vi "DANTE acquire single.vi"(0 "Acq in progress":refnum<vi>, 1 "Single Spectrum":refnum<vi>, 6 "Number of boards in chain":u8(slide)=1 scale=1.0..8.0, 8 "Pause button":refnum<vi>, 9 "Acquisition time [s]":dbl=10.0 min=1.0 max=1000.0, 10 "Stop Button":refnum<vi>, 11 "identifier out":string) -> (2 "stats out":T1, 3 "single spectrum":dbl[](array[numeric]))   [LabVIEW 2015]
uses:
  StateTypeDef.ctl
  XGL_DPP.lvlib
panel:
  in  "Stop Acq":bool
  out "Boards to configure":u8(slide) scale=0.0..8.0
  out "spectra to read 3":i64=10
  out "spectra to read":i64=1
  out "spectra":u16[][](array[numeric])
  out "adv stats":u64[][](array[numeric])
  out "Statistics":dbl[][](array[numeric])
  out "State 2":T2=enum."Close library"
  in  "Map points":u32=10
  in  "Time per spectrum [ms]":u32=10 min=1 max=1000000
  in  "Add IP":bool
  out "Acq. in progress":bool
  out "Library Initialized":bool
  in  "Get connected":bool
  in  "Init":bool
  in  "Clear":bool
  in  "Close":bool
  in  "Start acq":bool
  out "Error code":i32
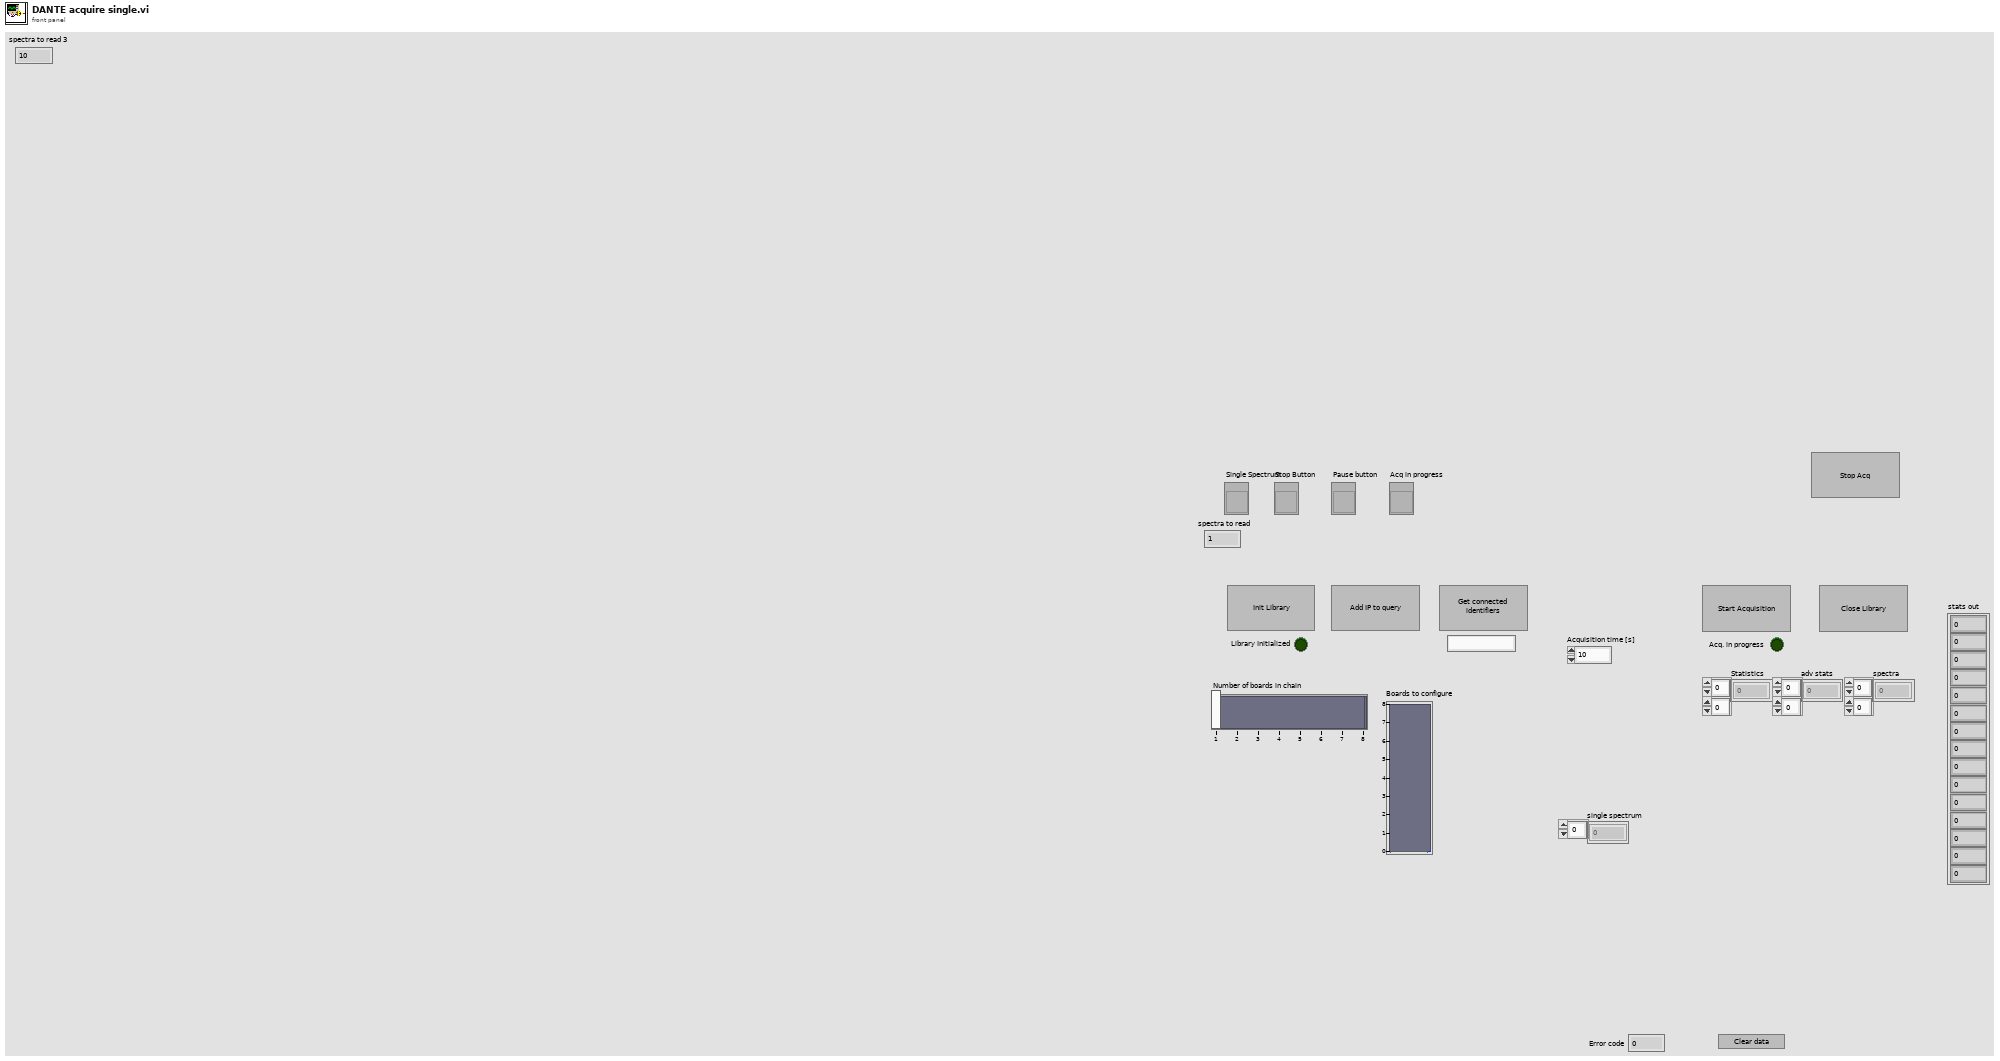
[diagram p1: front panel]
types:
  T1 = cluster{u64, u64, dbl, dbl, u32, u32, u32, u32, u32, u32, u32, u32, u32, u32, u32}
  T2 = typedef "StateTypeDef.ctl" = enum16{"Stop", "Check downloaded spectra", "Get all data", "Read acq mode", "Send running/Get Data", "Add IP to query", "Get serial", "Close library", "Clear", "Acquisition start", "Initialization", "Check Answer", "Configuring", "Wait Answer", "Start map", "Wait input"}
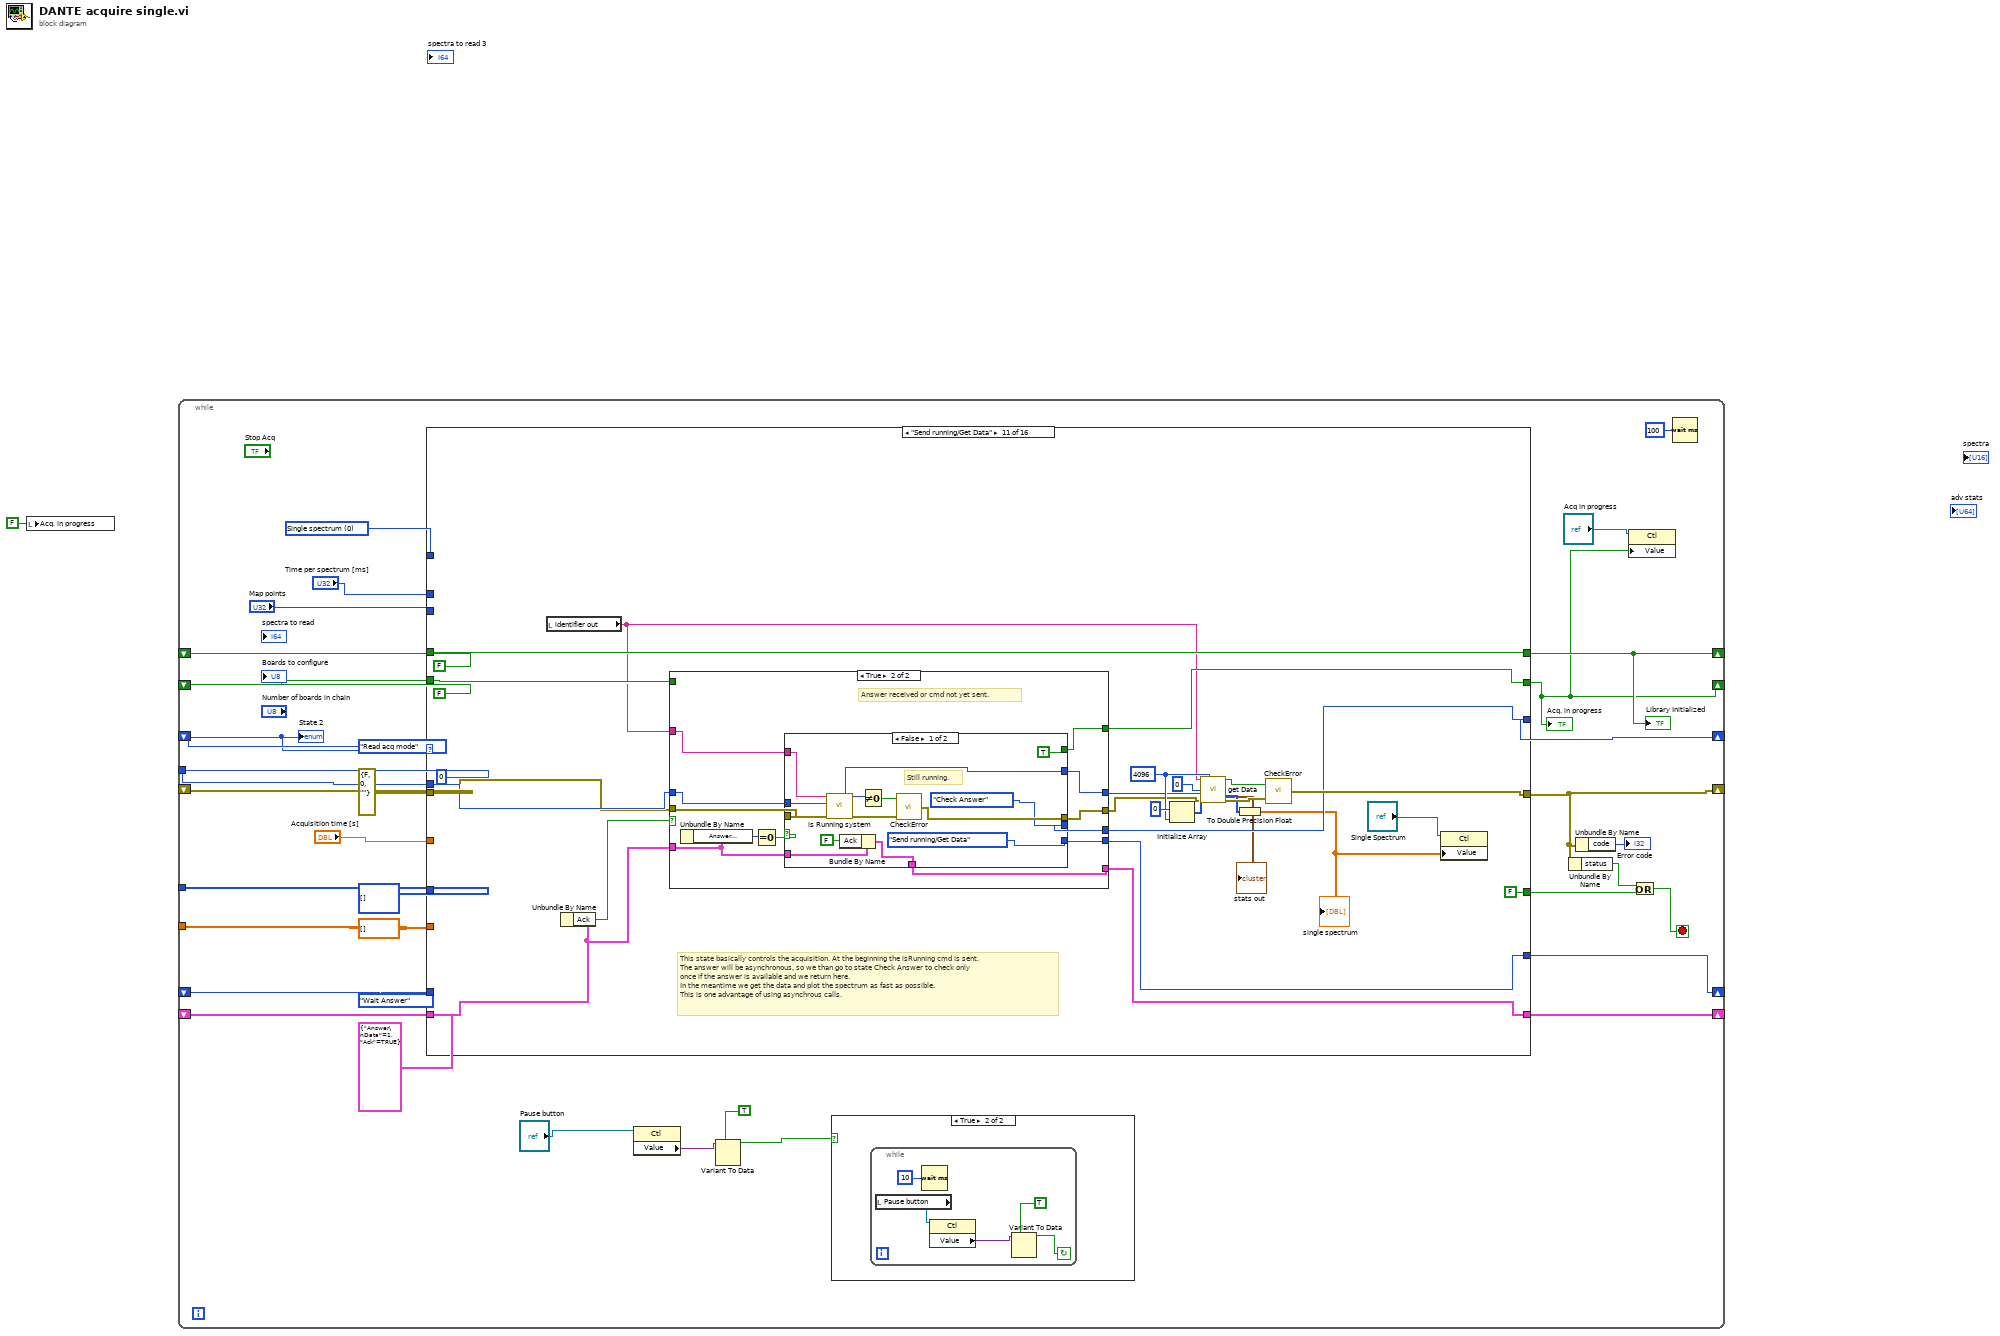
[diagram p0: block diagram]
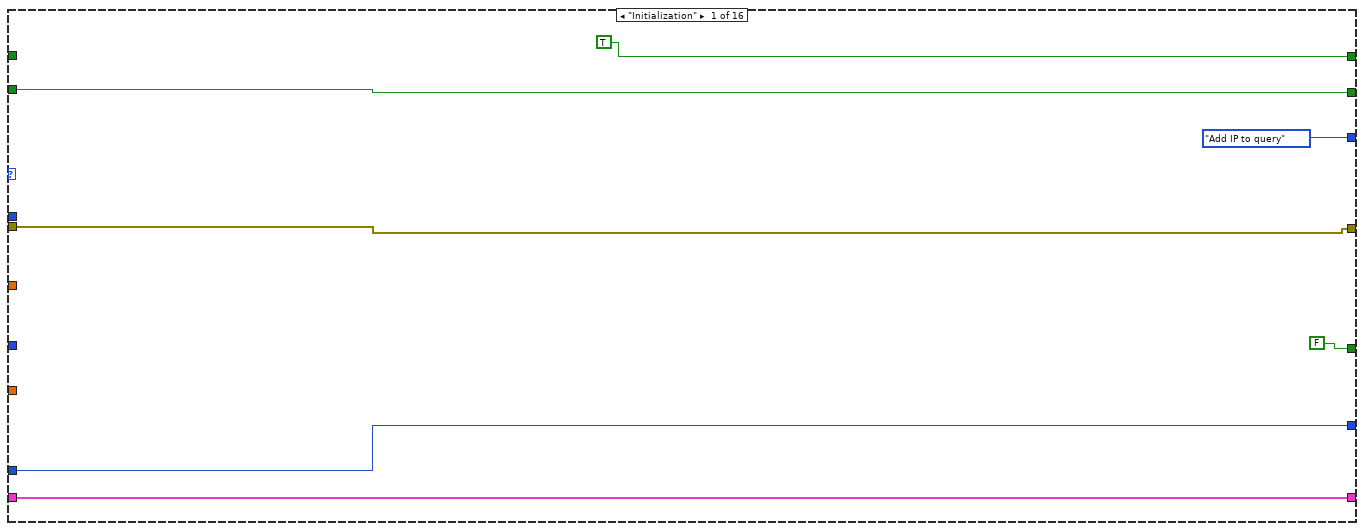
[diagram p3: hidden frame]
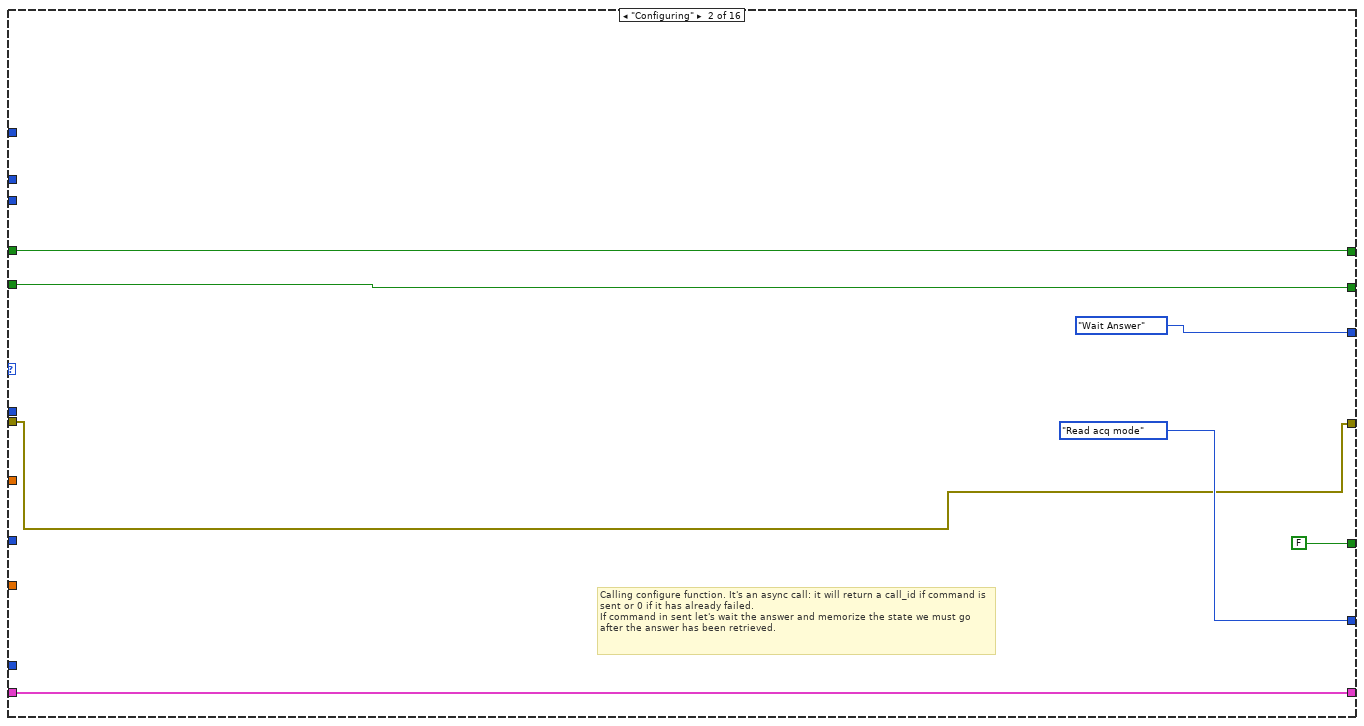
[diagram p4: hidden frame]
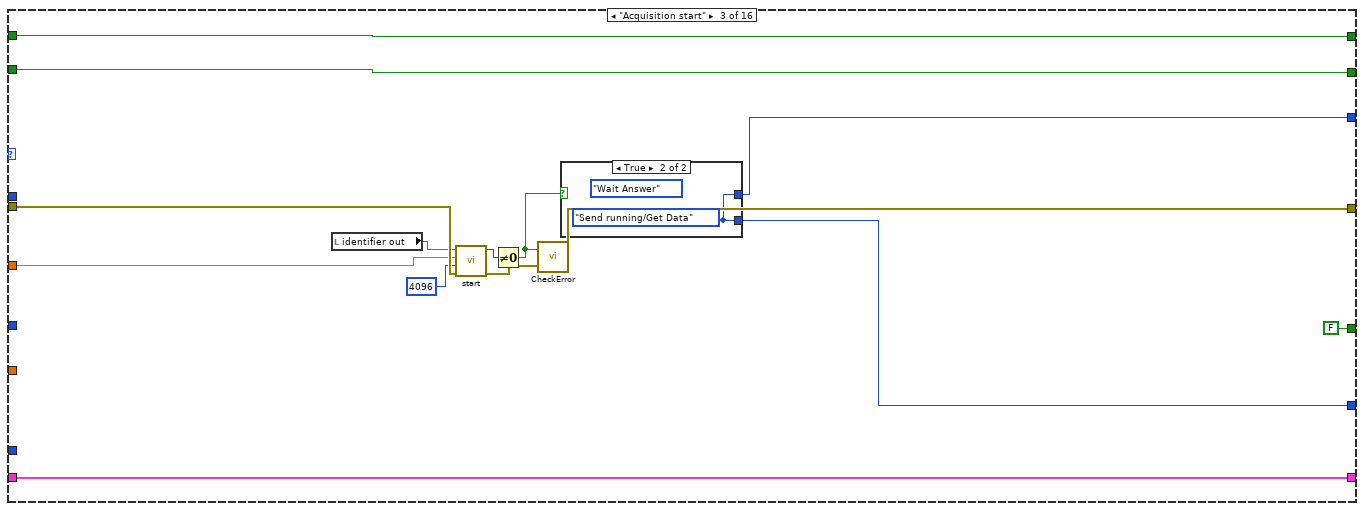
[diagram p5: hidden frame]
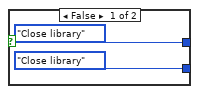
[diagram p6: hidden frame]
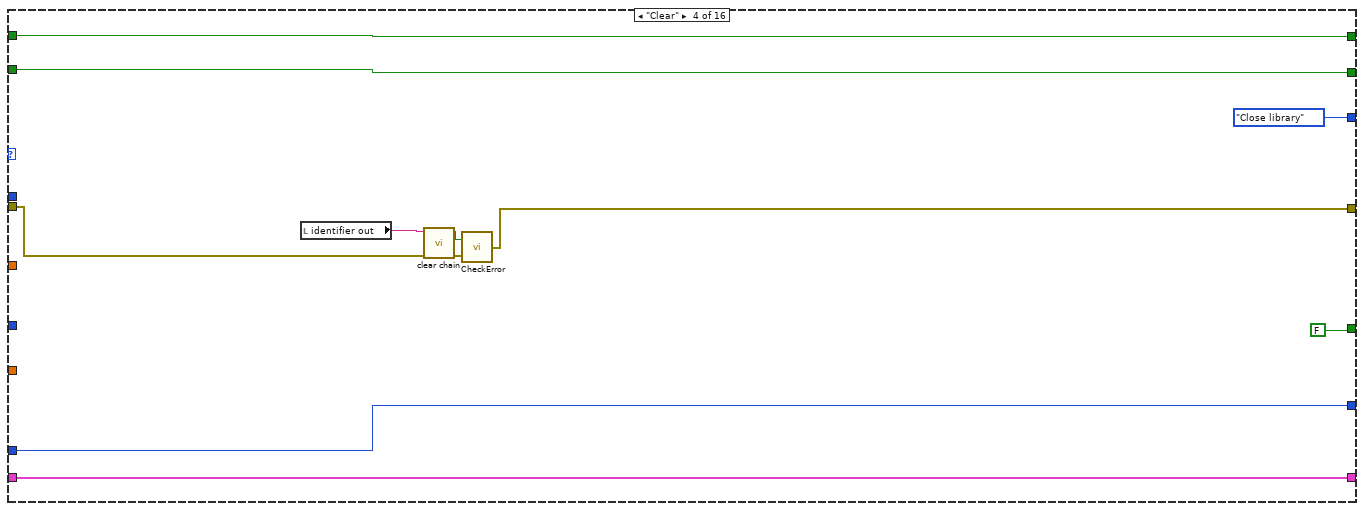
[diagram p7: hidden frame]
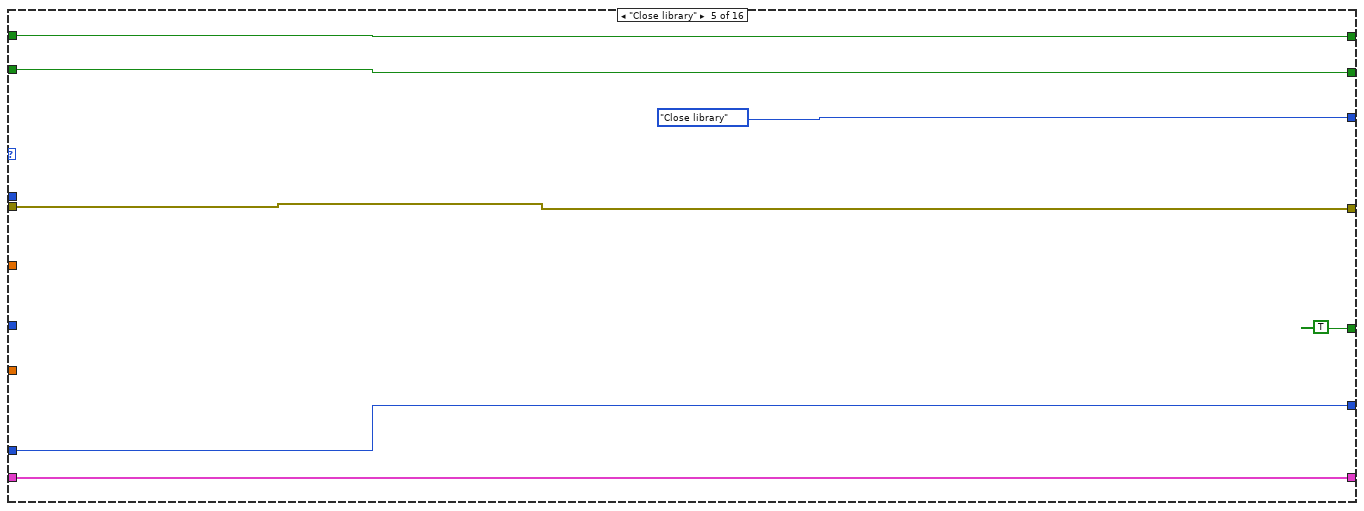
[diagram p8: hidden frame]
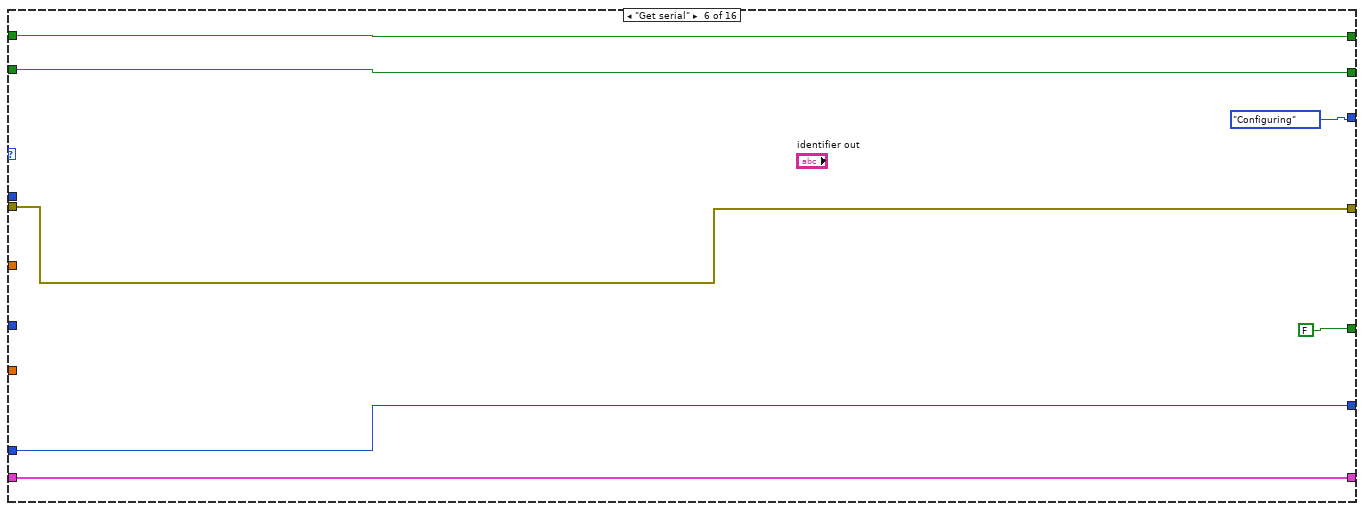
[diagram p9: hidden frame]
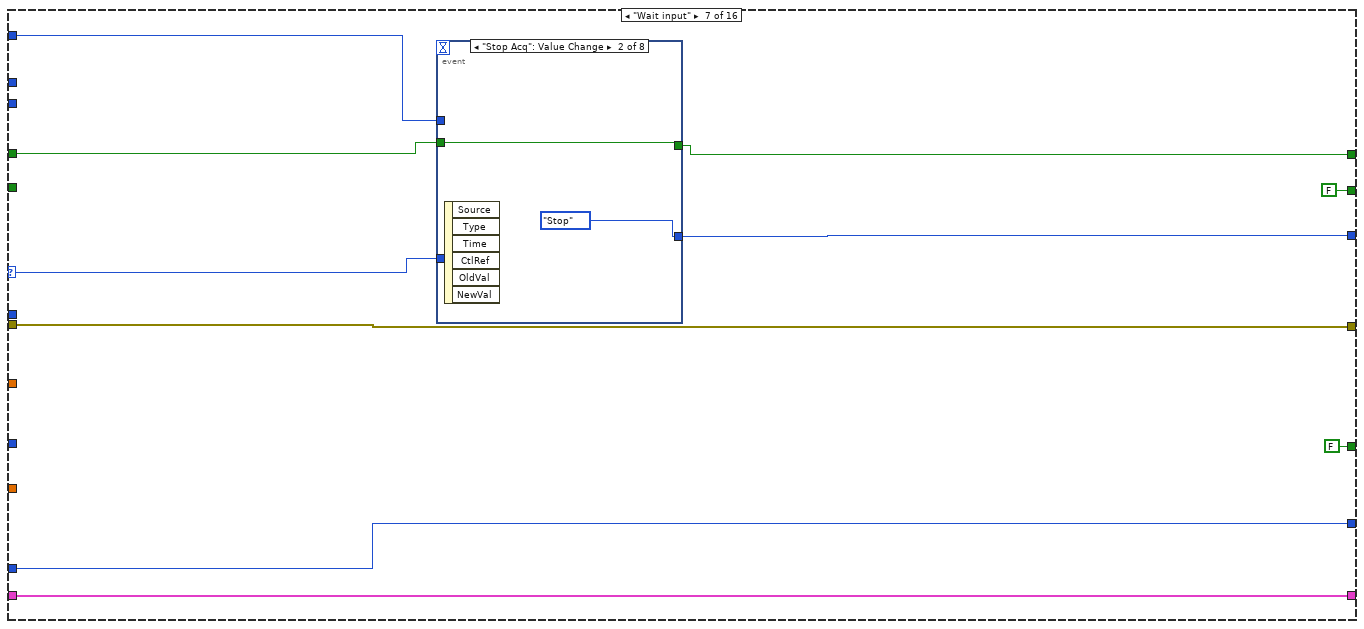
[diagram p10: hidden frame]
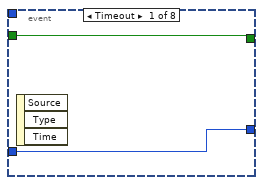
[diagram p11: hidden frame]
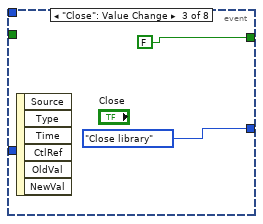
[diagram p12: hidden frame]
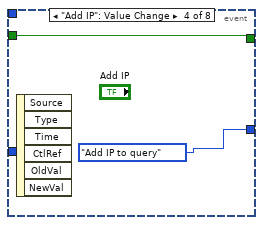
[diagram p13: hidden frame]
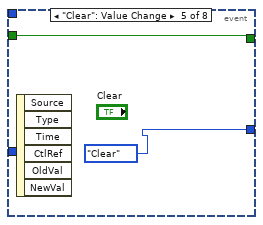
[diagram p14: hidden frame]
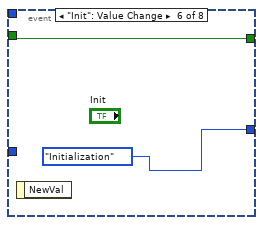
[diagram p15: hidden frame]
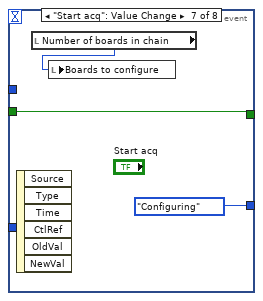
[diagram p16: hidden frame]
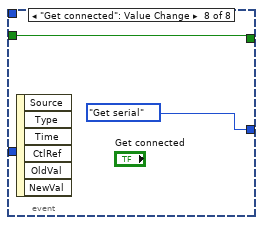
[diagram p17: hidden frame]
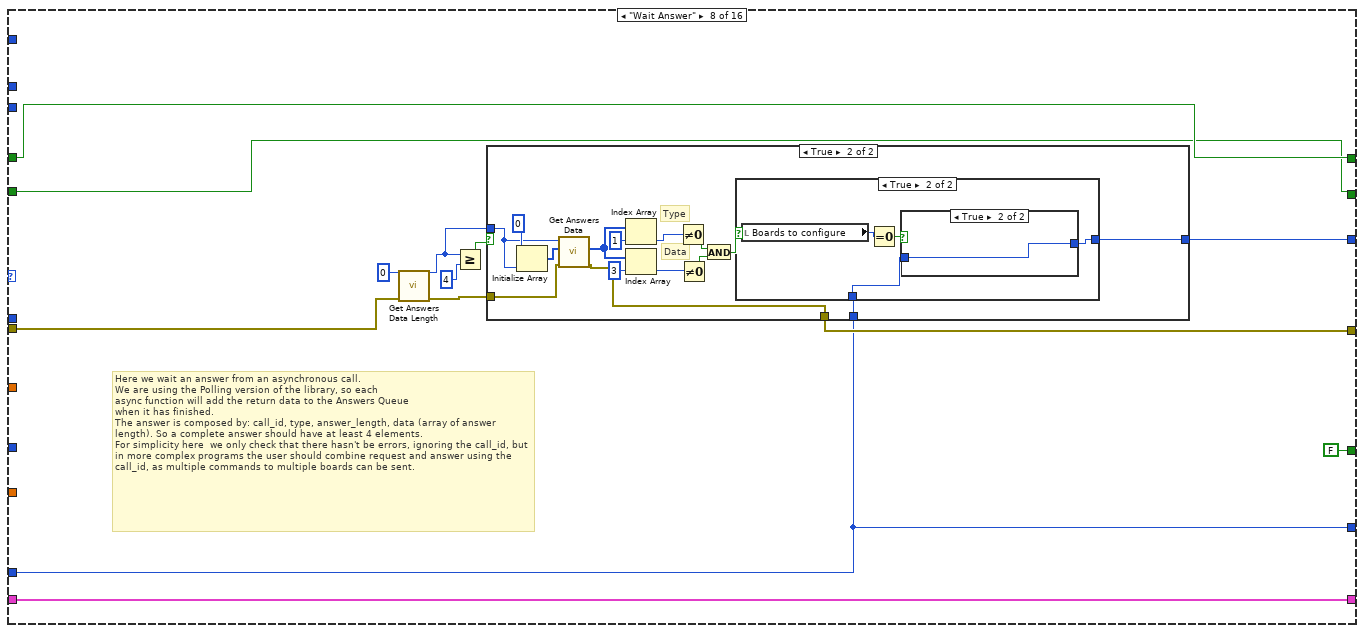
[diagram p18: hidden frame]
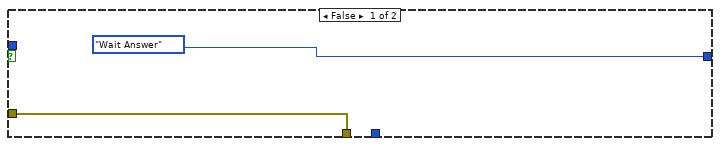
[diagram p19: hidden frame]
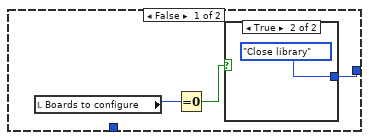
[diagram p20: hidden frame]
diagram:
  n1 = local write "Acq. in progress"(FALSE ("Acq. in progress")) -> ()
  n2 = while {
    shift-right: [w37] -> _
    shift-left: errorcluster {"status"=FALSE, "code"=0, "source"=""} ("error in (no error)") -> [w39]
    shift-right: [w26] -> _
    shift-left: StateTypeDef."Read acq mode" ("State") -> [w22]
    shift-right: [w31] -> _
    shift-left: FALSE -> [w32]
    shift-right: [w11] -> _
    shift-left: FALSE -> [w30]
    tunnel: u16 0 ("Board") -> [w29]
    shift-right: [w28] -> _
    shift-left: StateTypeDef."Wait Answer" ("State") -> [w27]
    shift-right: [w24] -> _
    shift-left: cluster{"Answer\nData":i32, "Ack":bool} {"Answer\nData"=1, "Ack"=TRUE} -> [w25]
    tunnel: dbl[] [] ("Y") -> [w18]
    tunnel: u16[][] [] ("element") -> [w17]
    stop <- w35 stop-if-true
    w23 = u16 0 items=["Single spectrum", "Multiple spectra"] ("Acquisition mode")
    n3 = case shown="\"Send running/Get Data\"" w22 {
      selector: w22 -> [_ _ _ _ _ _ w109 _ _ _ _ _ _ _ _ _]
      tunnel: w39 -> [w45 w52 w70 w81 w87 w94 w108 w140 w184 w229 w259 w302 w323 w334 w402 w428]
      tunnel: [w45 w52 w64 w76 w87 w94 w108 w134 w171 w229 w258 w302 w320 w332 w402 w424] -> w37
      tunnel: [StateTypeDef."Add IP to query" ("State") StateTypeDef."Wait Answer" ("State") w68 StateTypeDef."Close library" ("State") StateTypeDef."Close library" ("State") StateTypeDef."Configuring" ("State") w110 w130 w173 StateTypeDef."Get serial" ("State") w253 w305 w319 StateTypeDef."Check downloaded spectra" ("State") w404 StateTypeDef."Wait Answer" ("State")] -> w26
      tunnel: "Acquisition time [s]" -> [_ _ w69 _ _ _ _ _ _ _ _ _ _ _ _ _]
      tunnel: [FALSE ("y") FALSE ("y") FALSE ("y") FALSE ("y") TRUE ("y") FALSE ("y") FALSE ("y") FALSE ("y") FALSE ("y") FALSE ("y") FALSE ("y") FALSE FALSE FALSE FALSE TRUE] -> w33
      tunnel: [TRUE w57 w72 w85 w92 w99 w106 w132 w182 w235 w257 w304 w317 w336 w403 w419] -> w31
      tunnel: w32 -> [_ w57 w72 w85 w92 w99 w105 w132 w182 w235 w257 w304 w317 w336 w403 w419]
      tunnel: [w50 w56 w71 w84 w91 w98 FALSE w131 w181 w234 w251 w303 w316 w337 w391 FALSE] -> w11
      tunnel: w30 -> [w50 w56 w71 w84 w91 w98 _ w131 w181 w234 w250 w303 w316 _ _ _]
      tunnel: w29 -> [_ _ _ _ _ _ _ _ _ _ w260 _ _ _ _ _]
      tunnel: [w49 StateTypeDef."Read acq mode" ("State") w66 w83 w90 w97 w104 w129 w175 w233 w254 w305 w318 w338 w400 StateTypeDef."Get all data" ("State")] -> w28
      tunnel: w27 -> [w49 _ _ w83 w90 w97 w104 w129 w176 w233 _ _ _ w338 w400 _]
      tunnel: w25 -> [w48 w53 w63 w82 w89 w96 w103 w128 w183 w231 w256 w300 w314 w339 w399 w421]
      tunnel: [w48 w53 w63 w82 w89 w96 w103 w128 w177 w231 w255 w300 w314 w339 w399 w421] -> w24
      tunnel: w23 -> [_ _ _ _ _ _ w102 _ _ _ _ w306 _ _ _ _]
      tunnel: "Time per spectrum [ms]" -> [_ _ _ _ _ _ _ _ _ _ _ _ w324 _ w398 _]
      tunnel: "Map points" -> [_ _ _ _ _ _ _ _ _ _ _ _ w311 _ _ _]
      tunnel: w17 -> [_ _ _ _ _ _ _ _ _ _ _ _ _ _ _ _]
      tunnel: w18 -> [_ _ _ _ _ _ _ _ _ _ _ _ _ _ _ _]
      frame "Initialization" {
      }
      frame "Configuring" {
        # "Calling configure function. It's an async call: it will return a call_id if command is sent or 0 if it has already failed.\nIf command in sent let's wait the answer and memorize the state we must go after the answer has been retrieved."
      }
      frame "Acquisition start" {
        n4 = local read "identifier out"() -> (w60:string)
        n5 = call "start.vi"("error in (no error)"=w70, "spect_depth"=u16 4096, "time"=w69, "identifier"=w60) -> ("error out"=w65:errorcluster, "function return"=w62:u32)  [unwired: 6 in]
        n6 = Not Equal To 0?(x=w62) -> (x != 0?=w61:bool)
        n7 = call "CheckError.vi"("error in (no error)"=w65, "ret_val"=w61) -> ("error out"=w64:errorcluster)
        n8 = case shown="True" w61 {
          tunnel: [StateTypeDef."Close library" ("State") w75] -> w68
          tunnel: [StateTypeDef."Close library" ("State") w75] -> w66
          frame False {
          }
          frame True {
            w75 = StateTypeDef."Send running/Get Data" ("State")
            (unwired) StateTypeDef."Wait Answer" ("State")
          }
        }
      }
      frame "Clear" {
        n9 = local read "identifier out"() -> (w77:string)
        n10 = call "clear chain.vi"("error in (no error)"=w81, "identifier"=w77) -> ("error out"=w79:errorcluster, "function return"=w80:bool)  [unwired: 8 in]
        n11 = call "CheckError.vi"("error in (no error)"=w79, "ret_val"=w80) -> ("error out"=w76:errorcluster)
      }
      frame "Close library" {
      }
      frame "Get serial" {
      }
      frame "Wait input" {
        n12 = event shown="[1] \"Stop Acq\": Value Change" {
          selector: _ -> [_ _ _ _ _ _ _ _]
          dyn-events: _ -> [_ _ _ _ _ _ _ _]
          timeout: _ -> [_ _ _ _ _ _ _ _]
          tunnel: [w112 StateTypeDef."Stop" ("State") StateTypeDef."Close library" ("State") StateTypeDef."Add IP to query" ("State") StateTypeDef."Clear" ("State") StateTypeDef."Initialization" ("State") StateTypeDef."Configuring" ("State") StateTypeDef."Get serial" ("State")] -> w110
          tunnel: w109 -> [w112 _ _ _ _ _ _ _]
          tunnel: [w111 w113 FALSE w118 w120 w122 w125 w127] -> w106
          tunnel: w105 -> [w111 w113 _ w118 w120 w122 w125 w127]
          tunnel: w102 -> [_ _ _ _ _ _ _ _]
          event Timeout {
            n13 = event-data() -> ()  [unwired: 1 in, 3 out]
          }
          event "Stop Acq": Value Change {
            n14 = event-data() -> ()  [unwired: 1 in, 6 out]
          }
          event "Close": Value Change {
            n15 = event-data() -> ()  [unwired: 1 in, 6 out]
          }
          event "Add IP": Value Change {
            n16 = event-data() -> ()  [unwired: 1 in, 6 out]
          }
          event "Clear": Value Change {
            n17 = event-data() -> ()  [unwired: 1 in, 6 out]
          }
          event "Init": Value Change {
            n18 = event-data() -> ()  [unwired: 1 in, 1 out]
          }
          event "Start acq": Value Change {
            n19 = event-data() -> ()  [unwired: 1 in, 6 out]
            n20 = local read "Number of boards in chain"() -> (w123:u8)
            n21 = local write "Boards to configure"(w123) -> ()
          }
          event "Get connected": Value Change {
            n22 = event-data() -> ()  [unwired: 1 in, 6 out]
          }
        }
      }
      frame "Wait Answer" {
        # "Here we wait an answer from an asynchronous call.\nWe are using the Polling version of the library, so each\nasync function will add the return data to the Answers Queue\nwhen it has finished.\nThe answer is composed by: call_id, type, answer_length, data (array of answer length). So a complete answer should have at least 4 elements.\nFor simplicity here  we only check that there hasn't be errors, ignoring the call_id, but in more complex programs the user should combine request and answer using the call_id, as multiple commands to multiple boards can be sent."
        n23 = call "Get Answers Data Length.vi"("error in (no error)"=w140, "length"=u32 0) -> ("error out"=w136:errorcluster, "length out"=w135:u32)  [unwired: 7 in, 1 out]
        n24 = Greater Or Equal?(x=w135, y=u32 4) -> (x >= y?=w137:bool)
        n25 = case shown="True" w137 {
          tunnel: w136 -> [w142 w145]
          tunnel: w135 -> [_ w147]
          tunnel: w129 -> [_ w149]
          tunnel: [w142 w144] -> w134
          tunnel: [StateTypeDef."Wait Answer" ("State") w148] -> w130
          frame False {
          }
          frame True {
            # "Data"
            # "Type"
            n26 = Initialize Array(u32 0 ("y"), w147) -> (w146:u32[])
            n27 = call "Get Answers Data.vi"("error in (no error)"=w145, "data"=w146, "length"=w147) -> ("error out"=w144:errorcluster, "data out"=w143:u32[])  [unwired: 4 in, 1 out]
            n28 = Index Array(array=w143, index=1) -> (element=w153:u32)
            n29 = Index Array(array=w143, index=3) -> (element=w154:u32)
            n30 = Not Equal To 0?(x=w153) -> (x != 0?=w151:bool)
            n31 = Not Equal To 0?(x=w154) -> (x != 0?=w152:bool)
            n32 = And(x=w151, y=w152) -> (x .and. y?=w150:bool)
            n33 = case shown="True" w150 {
              tunnel: w149 -> [_ w163]
              tunnel: [w160 w164] -> w148
              frame False {
                n34 = local read "Boards to configure"() -> (w159:u8)
                n35 = Equal To 0?(x=w159) -> (x = 0?=w158:bool)
                n36 = case shown="True" w158 {
                  tunnel: [StateTypeDef."Configuring" ("State") StateTypeDef."Close library" ("State")] -> w160
                  frame False {
                  }
                  frame True {
                  }
                }
              }
              frame True {
                n37 = local read "Boards to configure"() -> (w166:u8)
                n38 = Equal To 0?(x=w166) -> (x = 0?=w165:bool)
                n39 = case shown="True" w165 {
                  tunnel: [StateTypeDef."Configuring" ("State") w168] -> w164
                  tunnel: w163 -> [_ w168]
                  frame False {
                  }
                  frame True {
                  }
                }
              }
            }
          }
        }
      }
      frame "Check Answer" {
        # "Here I check if an answer is available. If it is, I pass the data to a variable.\nThen I return to the 'next state' in any case, even if no answer is yet available."
        n40 = call "Get Answers Data Length.vi"("error in (no error)"=w184, "length"=u32 0) -> ("error out"=w186:errorcluster, "length out"=w185:u32)  [unwired: 7 in, 1 out]
        n41 = Greater Or Equal?(x=w185, y=u32 4) -> (x >= y?=w187:bool)
        n42 = case shown="True" w187 {
          tunnel: w186 -> [w201 w206]
          tunnel: w185 -> [_ w204]
          tunnel: [w201 w212] -> w172
          tunnel: [w200 w211] -> w174
          tunnel: w176 -> [w200 w210]
          tunnel: w183 -> [w199 w208]
          tunnel: [w199 w209] -> w178
          frame False {
            # "Do not update answer data."
          }
          frame True {
            # "Data"
            # "Type"
            n43 = Initialize Array(u32 0 ("y"), w204) -> (w203:u32[])
            n44 = call "Get Answers Data.vi"("error in (no error)"=w206, "data"=w203, "length"=w204) -> ("error out"=w205:errorcluster, "data out"=w202:u32[])  [unwired: 4 in, 1 out]
            n45 = Index Array(array=w202, index=1) -> (element=w214:u32)
            n46 = Index Array(array=w202, index=3) -> (element=w207:u32)
            n47 = Not Equal To 0?(x=w214) -> (x != 0?=w213:bool)
            n48 = case shown="False" w213 {
              selector: w213 -> [w222 w224]
              tunnel: w205 -> [w221 w228]
              tunnel: [w220 w228] -> w212
              tunnel: [StateTypeDef."Close library" ("State") w227] -> w211
              tunnel: w210 -> [_ w227]
              tunnel: [w219 w225] -> w209
              tunnel: w208 -> [w219 w226]
              tunnel: w207 -> [_ w223]
              frame False {
                # "Type = 0, an error occurred."
                n49 = call "CheckError.vi"("error in (no error)"=w221, "ret_val"=w222) -> ("error out"=w220:errorcluster)
              }
              frame True {
                # "Type 1 or 2, which means\nanswer of a read or write cmd."
                n50 = Bundle By Name(cluster=w226, "Answer\nData"=w223, "Ack"=w224) -> (w225:cluster{"Answer\nData":i32, "Ack":bool})
              }
            }
          }
        }
        n51 = property on="Property Node" class="Ctl"(reference="Stop Button") -> ("Value"=w180:variant)  [unwired: 1 in, 2 out]
        n52 = Variant To Data(type=TRUE, Variant=w180) -> (data=w170:bool)  [unwired: 1 in, 1 out]
        n53 = case shown="True" w170 {
          tunnel: w178 -> [w191 w198]
          tunnel: [w191 w198] -> w177
          tunnel: w176 -> [w192 _]
          tunnel: [w192 StateTypeDef."Stop" ("State")] -> w175
          tunnel: w174 -> [w194 _]
          tunnel: [w194 StateTypeDef."Stop" ("State")] -> w173
          tunnel: w172 -> [w193 w195]
          tunnel: [w193 w195] -> w171
          frame False {
          }
          frame True {
          }
        }
      }
      frame "Add IP to query" {
      }
      frame "Send running/Get Data" {
        w246 = u32 4096 ("spectra_size")
        # "This state basically controls the acquisition. At the beginning the isRunning cmd is sent.\nThe answer will be asynchronous, so we than go to state Check Answer to check only\nonce if the answer is available and we return here.\nIn the meantime we get the data and plot the spectrum as fast as possible.\nThis is one advantage of using asynchrous calls."
        n54 = local read "identifier out"() -> (w240:string)
        n55 = Unbundle By Name(w256) -> ("Ack"=w249:bool)
        n56 = case shown="True" w249 {
          tunnel: w260 -> [w266 w273]
          tunnel: w259 -> [w265 w274]
          tunnel: [w265 w272] -> w242
          tunnel: [w266 w271] -> w241
          tunnel: w256 -> [w264 w276]
          tunnel: [w264 w275] -> w255
          tunnel: [StateTypeDef."Send running/Get Data" ("State") w270] -> w254
          tunnel: [StateTypeDef."Check Answer" ("State") w269] -> w253
          tunnel: [w263 w268] -> w251
          tunnel: w250 -> [w263 _]
          tunnel: w240 -> [_ w267]
          frame False {
            # "Command sent, wait the answer before\nsending another command."
          }
          frame True {
            # "Answer received or cmd not yet sent."
            n57 = Unbundle By Name(w276) -> ("Answer\nData"=w278:i32)
            n58 = Equal To 0?(x=w278) -> (x = 0?=w277:bool)
            n59 = case shown="False" w277 {
              tunnel: [StateTypeDef."Send running/Get Data" ("State") w292] -> w270
              tunnel: [StateTypeDef."Check Answer" ("State") w292] -> w269
              tunnel: w276 -> [w288 w299]
              tunnel: [w287 w296] -> w275
              tunnel: w274 -> [w291 w294]
              tunnel: w273 -> [w285 w295]
              tunnel: [w289 w294] -> w272
              tunnel: [w285 w295] -> w271
              tunnel: [TRUE FALSE] -> w268
              tunnel: w267 -> [w279 _]
              frame False {
                # "Still running."
                n60 = call "is Running system.vi"("error in (no error)"=w291, "Board"=w285, "identifier"=w279) -> ("error out"=w290:errorcluster, "function return"=w282:u32)  [unwired: 7 in]
                n61 = Bundle By Name(cluster=w288, "Ack"=FALSE) -> (w287:cluster{"Answer\nData":i32, "Ack":bool})
                n62 = Not Equal To 0?(x=w282) -> (x != 0?=w283:bool)
                n63 = call "CheckError.vi"("error in (no error)"=w290, "ret_val"=w283) -> ("error out"=w289:errorcluster)
              }
              frame True {
                w292 = StateTypeDef."Close library" ("State")
                # "Board has finished acquisition."
                n64 = Bundle By Name(cluster=w299, "Answer\nData"=1 ("Answer\nData"), "Ack"=TRUE) -> (w296:cluster{"Answer\nData":i32, "Ack":bool})
              }
            }
          }
        }
        n65 = Initialize Array(u64 0 ("acq_status"), w246) -> (w245:u64[])
        n66 = call "get Data.vi"("identifier"=w240, "spectra_size"=w246, "Board"=w241, "id"=u32 0, "values"=w245, "error in (no error)"=w242) -> ("function return"=w243:bool, "values out"=w239:u64[], "stats out"=→"stats out":T1, "error out"=w244:errorcluster)  [unwired: 5 in, 1 out]
        n67 = To Double Precision Float(number=w239) -> (double precision float=w236:dbl[])
        "single spectrum" <- w236
        n68 = call "CheckError.vi"("error in (no error)"=w244, "ret_val"=w243) -> ("error out"=w258:errorcluster)
        n69 = property on="Property Node" class="Ctl"(reference="Single Spectrum", "Value"=w236) -> ()  [unwired: 1 in, 2 out]
      }
      frame "Read acq mode" {
        # "Start issued. Check the selected acquisition mode."
        n70 = case shown="0, Default" w306 {
          tunnel: [StateTypeDef."Acquisition start" ("State") StateTypeDef."Start map" ("State")] -> w305
          frame 0, Default {
          }
          frame 1 {
          }
        }
      }
      frame "Start map" {
        n71 = local read "Number of boards in chain"() -> (w310:u8)
        n72 = local read "identifier out"() -> (w313:string)
        n73 = Multiply(x=w311, y=w310) -> (x*y=w312:u32)
        n74 = local write "spectra to read"(w312) -> ()
        n75 = call "start map.vi"("spect_depth"=u16 4096, "error in (no error)"=w323, "points"=w311, "sp_time"=w324, "identifier"=w313) -> ("error out"=w322:errorcluster, "function return"=w321:u32)  [unwired: 5 in]
        n76 = Not Equal To 0?(x=w321) -> (x != 0?=w325:bool)
        n77 = call "CheckError.vi"("error in (no error)"=w322, "ret_val"=w325) -> ("error out"=w320:errorcluster)
        n78 = case shown="True" w325 {
          tunnel: [StateTypeDef."Close library" ("State") StateTypeDef."Wait Answer" ("State")] -> w319
          tunnel: [StateTypeDef."Close library" ("State") StateTypeDef."Get all data" ("State")] -> w318
          frame False {
          }
          frame True {
          }
        }
      }
      frame "Get all data" {
        # "Get the nb of spectra available and if greater than 0 get them.\nThe spectrum and statistics are returned as 1D arrays (one append to the other)\nso they are reshaped as 2D arrays.\nIn this example all the spectra are stored in a 2D array, that at the end of the measure \nwill have dimensions nb_spectra x 4096. Statistics are just reshaped but not used."
        n79 = local read "Number of boards in chain"() -> (w330:u8)
        n80 = local read "identifier out"() -> (w333:string)
        n81 = for {
          N: w330 -> [_]
          tunnel: [TRUE] -> w337
          tunnel: w333 -> [w346]
          shift-right: [w341] -> w332
          shift-left: w334 -> [w348]
          i -> [w340]
          n82 = call "get Available Data.vi"("error in (no error)"=w348, "Board"=w340, "identifier"=w346) -> ("error out"=w363:errorcluster, "data_number out"=w349:u32, "function return"=w364:bool)  [unwired: 6 in]
          n83 = Greater Than 0?(x=w349) -> (x > 0?=w362:bool)
          n84 = call "CheckError.vi"("error in (no error)"=w363, "ret_val"=w364) -> ("error out"=w361:errorcluster)
          n85 = Multiply(x=w349, y=u32 4096) -> (x*y=w356:u32)
          n86 = Multiply(x=w349, y=u32 4) -> (x*y=w353:u32)
          n87 = Multiply(x=w349, y=u32 24) -> (x*y=w350:u32)
          n88 = Initialize Array(u32 0, w349) -> (w347:u32[])
          n89 = Initialize Array(u16 0, w356) -> (w345:u16[])
          n90 = Initialize Array(0.0, w353) -> (w344:dbl[])
          n91 = Initialize Array(u64 0, w350) -> (w343:u64[])
          n92 = case shown="False" w362 {
            tunnel: w340 -> [_ w374]
            tunnel: w361 -> [w365 w371]
            tunnel: [w365 w385] -> w341
            tunnel: w346 -> [_ w381]
            tunnel: w349 -> [_ w367]
            tunnel: w347 -> [_ w373]
            tunnel: w345 -> [_ w372]
            tunnel: u32 4096 ("spectra_size") -> [_ w370]
            tunnel: w344 -> [_ w369]
            tunnel: w343 -> [_ w368]
            tunnel: w340 -> [_ _]
            frame False {
              # "No spectrum available."
            }
            frame True {
              # "Adv stats reshaped"
              # "Statistics reshaped"
              # "Spectra reshaped"
              n93 = call "get All Data.vi"("identifier"=w381, "data_number"=w367, "id"=w373, "values"=w372, "error in (no error)"=w371, "spectra_size"=w370, "Board"=w374, "stats"=w369, "advstats"=w368) -> ("advstats out"=w388:u64[], "stats out"=w389:dbl[], "function return"=w387:bool, "values out"=w390:u16[], "error out"=w386:errorcluster)  [unwired: 3 in, 3 out]
              n94 = call "CheckError.vi"("error in (no error)"=w386, "ret_val"=w387) -> ("error out"=w385:errorcluster)
              n95 = Reshape Array(w388, w367, 24 ("dimension size")) -> ()  [unwired: 1 out]
              n96 = Reshape Array(w389, w367, 4 ("dimension size")) -> (→"Statistics":dbl[][])
              n97 = Reshape Array(w390, w367, u16 4096 ("dimension size")) -> (w366:u16[][])
              n98 = local read "spectra to read"() -> (w377:i64)
              n99 = Array Size(array=w366) -> (size(s)=w379:i32[])
              n100 = Index Array(array=w379, index=0) -> (element=w376:i32)
              n101 = Subtract(x=w377, y=w376) -> (x-y=w375:i64)
              n102 = local write "spectra to read"(w375) -> ()
            }
          }
        }
      }
      frame "Check downloaded spectra" {
        # "Check the current dimension of spectra 2D array. There can be this cases:\n- Downloaded spectra less than total_spectra-1 -> acquisition still in progress.\n- Down spectra equals total_spectra-1 ->acquisition almost finished, send stop.\nNote that the last spectrum will become available after the stop is sent. This because\nthe DLL mark as complete a spectrum if another spectrum arrives or the stop is issued.\n- Down spectra equals total_spectra -> acquisition finished, return to Wait Input."
        n103 = local read "Number of boards in chain"() -> (w392:u8)
        n104 = local read "spectra to read"() -> (w394:i64)
        n105 = Divide(x=w394, y=w392) -> (x/y=w393:dbl)
        n106 = Decrement(x=w393) -> (x-1=w397:dbl)
        n107 = Less Or Equal?(x=w397, y=u32 0) -> (x <= y?=w395:bool)
        n108 = case shown="False" w395 {
          tunnel: [StateTypeDef."Get all data" ("State") w411] -> w404
          tunnel: w398 -> [_ w410]
          tunnel: w397 -> [_ w409]
          tunnel: [TRUE w407] -> w391
          frame False {
          }
          frame True {
            n109 = Equal To 0?(x=w409) -> (x = 0?=w408:bool)
            n110 = case shown="False" w408 {
              tunnel: [StateTypeDef."Stop" ("State") StateTypeDef."Close library" ("State")] -> w411
              tunnel: w410 -> [w413 _]
              tunnel: [TRUE FALSE] -> w407
              frame True {
                n111 = Wait (ms)(milliseconds to wait=w413) -> ()  [unwired: 1 out]
              }
              frame False {
              }
            }
          }
        }
      }
      frame "Stop" {
        n112 = local read "identifier out"() -> (w417:string)
        n113 = call "stop.vi"("error in (no error)"=w428, "identifier"=w417) -> ("error out"=w425:errorcluster, "function return"=w427:u32)  [unwired: 8 in]
        n114 = Not Equal To 0?(x=w427) -> (x != 0?=w426:bool)
        n115 = call "CheckError.vi"("error in (no error)"=w425, "ret_val"=w426) -> ("error out"=w424:errorcluster)
      }
    }
    "Library Initialized" <- w31
    "Acq. in progress" <- w11
    n116 = property on="Property Node" class="Ctl"(reference="Pause button") -> ("Value"=w16:variant)  [unwired: 1 in, 2 out]
    n117 = Variant To Data(type=TRUE, Variant=w16) -> (data=w13:bool)  [unwired: 1 in, 1 out]
    n118 = case shown="True" w13 {
      frame False {
      }
      frame True {
        n119 = while {
          stop <- w40 continue-if-true
          n120 = local read "Pause button"() -> (w41:refnum<vi>)
          n121 = Wait (ms)(milliseconds to wait=u32 10) -> ()  [unwired: 1 out]
          n122 = property on="Property Node" class="Ctl"(reference=w41) -> ("Value"=w43:variant)  [unwired: 1 in, 2 out]
          n123 = Variant To Data(type=TRUE, Variant=w43) -> (data=w40:bool)  [unwired: 1 in, 1 out]
        }
      }
    }
    n124 = Unbundle By Name(w37) -> ("status"=w34:bool)
    n125 = Unbundle By Name(w37) -> ("code"=→"Error code":i32)
    n126 = property on="Property Node" class="Ctl"(reference="Acq in progress", "Value"=w11) -> ()  [unwired: 1 in, 2 out]
    n127 = Or(x=w34, y=w33) -> (x .or. y?=w35:bool)
    n128 = Wait (ms)(milliseconds to wait=u32 100) -> ()  [unwired: 1 out]
    "State 2" <- w22
  }
